vi "Set System Channel Properties.vi"(8 "error in (no error)":errorcluster, 9 "Channel Name":string, 10 "Channel Properties":cluster{"Name":string, "Value":variant}[](array[cluster]), 11 "tdms file in":refnum<k34>) -> (0 "error out":errorcluster, 3 "tdms file out":refnum<k34>)   [LabVIEW 2020, in "Telemetry Engine.lvlib"]
uses:
  Telemetry Engine.lvlib
  Shared/Constants.vi
  Shared/Telemetry Shared.lvlib
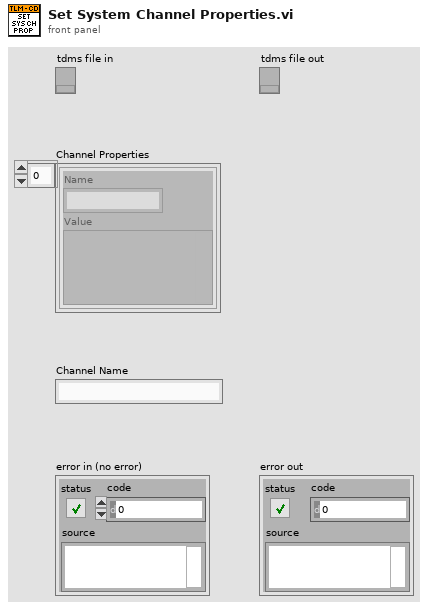
[diagram p1: front panel]
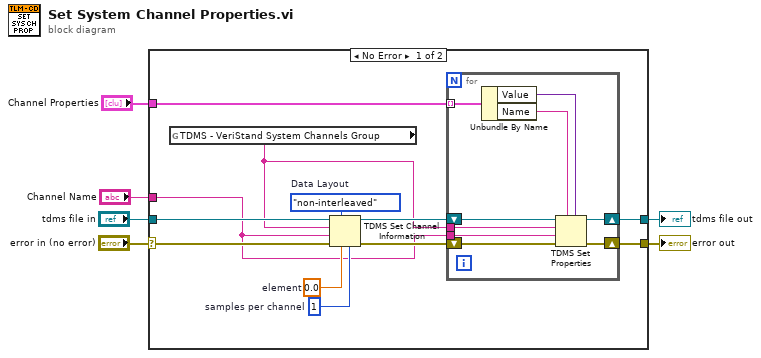
[diagram p0: block diagram]
diagram:
  n1 = case shown="No Error" "error in (no error)" {
    selector: "error in (no error)" -> [w10 w29]
    tunnel: "tdms file in" -> [w13 w28]
    tunnel: [w12 w29] -> w5
    tunnel: [w11 w28] -> w4
    tunnel: "Channel Properties" -> [w8 _]
    tunnel: "Channel Name" -> [w9 _]
    frame No Error {
      w18 = u32 1  # samples per channel
      w17 = 0.0  # element
      w16 = enum16{"non-interleaved", "interleaved"}."non-interleaved"  # Data Layout
      n2 = global read "Constants.vi" "TDMS - VeriStand System Channels Group"() -> (w7:string)
      n3 = TDMS Set Channel Information(4:w18, 6:w17, 7:w16, 8:w10, 9:w9, 10:w7, 11:w13) -> (0:w14:errorcluster, 3:w15:refnum<k34>)
      n4 = for {
        tunnel: w7 -> [w27]
        shift-right: [w23] -> w11
        shift-left: w15 -> [w26]
        shift-right: [w24] -> w12
        shift-left: w14 -> [w25]
        tunnel: w9 -> [w22]
        tunnel: w8 -> [w21] mode=indexing
        n5 = Unbundle By Name(w21) -> ("Value"=w19:variant, "Name"=w20:string)
        n6 = TDMS Set Properties(5:w19, 7:w20, 8:w25, 9:w22, 10:w27, 11:w26) -> (0:w24:errorcluster, 3:w23:refnum<k34>)  [unwired: 2 out]
      }
    }
    frame Error {
    }
  }
  "error out" <- w5
  "tdms file out" <- w4
